vi "OffsetFromCentre.vi"(5 "RangeMax":dbl, 7 "RangeMin":dbl, 10 "Value":dbl) -> (1 "OffsetFromCentre":dbl, 2 "LocationInRange":dbl, 3 "In Range?":bool)   [LabVIEW 2016]
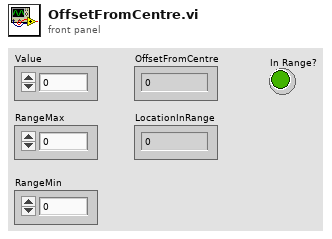
[diagram p1: front panel]
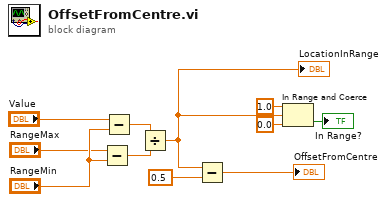
[diagram p0: block diagram]
diagram:
  n1 = Subtract(x="RangeMax", y="RangeMin") -> (x-y=w9:dbl)
  n2 = Subtract(x="Value", y="RangeMin") -> (x-y=w8:dbl)
  n3 = Divide(x=w8, y=w9) -> (x/y=w7:dbl)
  "LocationInRange" <- w7
  n4 = Subtract(x=w7, y=0.5) -> (x-y=→"OffsetFromCentre":dbl)
  n5 = In Range and Coerce(upper limit=1.0, x=w7, lower limit=0.0) -> (In Range?=→"In Range?":bool)  [unwired: 1 out]
